vi "importWaveform.vi"(2 "error in":errorcluster) -> (0 "error out":errorcluster, 1 "output waveform":waveform(dbl))   [LabVIEW 2023]
uses:
  <vilib>/Utility/file.llb/Read Delimited Spreadsheet (string).vi
panel:
  out "Waveform Graph":waveform(dbl)(graph)
  out "Window Type":string
  out "Pulse Duration":dbl
  out "End Freq":dbl
  out "Start Freq":dbl
  out "Sampling Rate":dbl
  in  "Path to Waveform":path
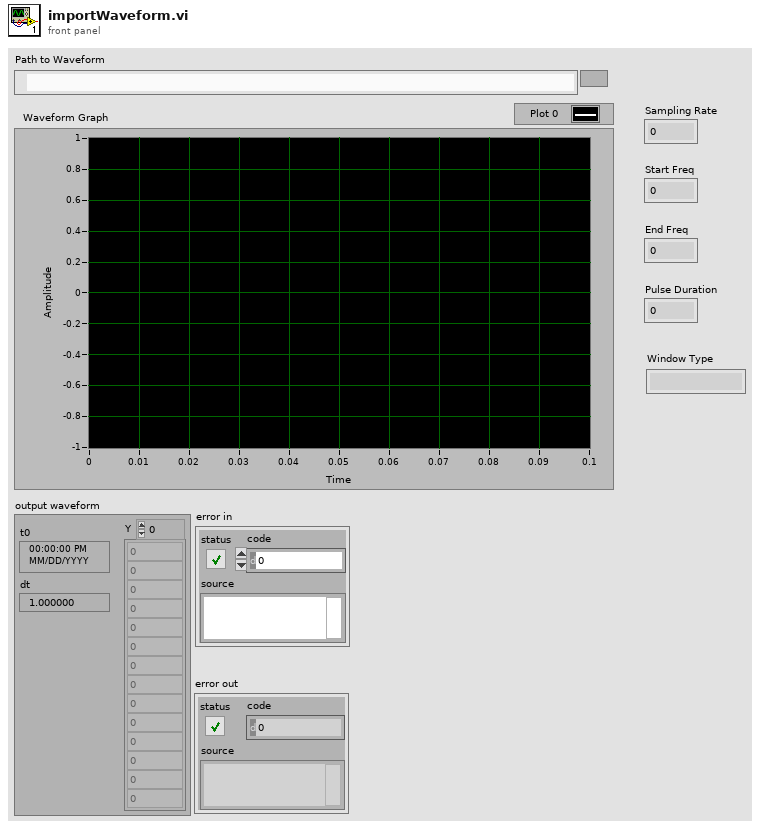
[diagram p1: front panel]
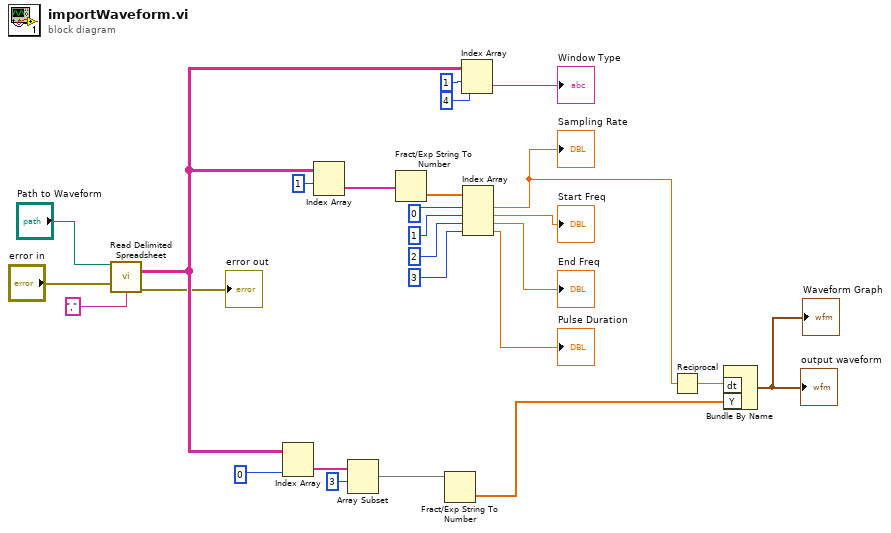
[diagram p0: block diagram]
diagram:
  n1 = call-poly <vilib>:"Read Delimited Spreadsheet.vi"("file path (dialog if empty)"="Path to Waveform", "error in (no error)"="error in", "delimiter (\\t)"="," ("delimiter (\\t)")) -> ("all rows"=w11:string[][], "error out"=→"error out":errorcluster)  [unwired: 7 in, 4 out]
  n2 = Index Array(array=w11, index (col)=0 ("disabled index (col)")) -> (element=w9:string[])  [unwired: 1 in]
  n3 = Index Array(array=w11, index (row)=1) -> (element=w15:string[])  [unwired: 1 in]
  n4 = Array Subset(array=w9, index=3) -> (w7:string[])  [unwired: 1 in]
  n5 = Fract/Exp String To Number(string=w15) -> (number=w23:dbl[])  [unwired: 3 in, 1 out]
  n6 = Fract/Exp String To Number(string=w7) -> (number=w4:dbl[])  [unwired: 3 in, 1 out]
  n7 = Index Array(array=w11, index (row)=1 ("index"), index (col)=4 ("disabled index (col)")) -> (element=→"Window Type":string)
  n8 = Index Array(array=w23, index #1=0 ("index"), index #2=1 ("index"), index #3=2 ("index"), index #4=3 ("index")) -> (element #1=w5:dbl, element #2=→"Start Freq":dbl, element #3=→"End Freq":dbl, element #4=→"Pulse Duration":dbl)
  "Sampling Rate" <- w5
  n9 = Reciprocal(x=w5) -> (1/x=w6:dbl)
  n10 = Bundle By Name("dt"=w6, "Y"=w4) -> (→"output waveform" →"Waveform Graph":waveform(dbl))  [unwired: 1 in]
